vi "HttpGet.vi"() -> ()   [LabVIEW 2016, in "wxpusher.lvlib"]
uses:
  wxpusher.lvlib
  <vilib>/httpClient/LabVIEWHTTPClient.lvlib
panel:
  out "body":string caption="体部"
  out "headers":string caption="头部"
  in  "error in":errorcluster caption="错误输入（无错误）"
  in  "指令+参数":string
  out "结果":string
  out "error out":errorcluster caption="错误输出"
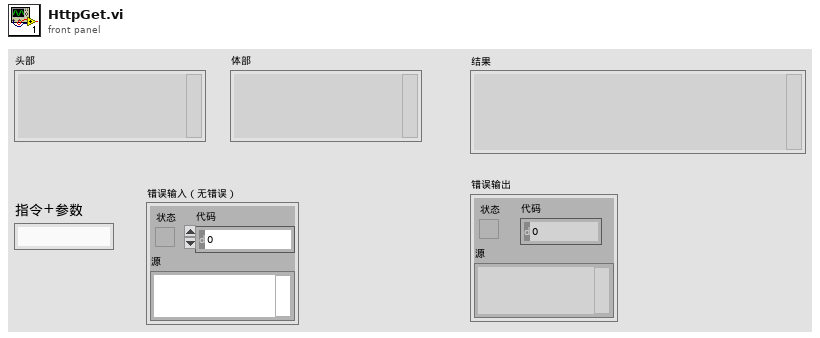
[diagram p1: front panel]
types:
  T1 = typedef "LabVIEWHTTPClient.lvlib/ClientHandle.ctl" = refnum<k1>
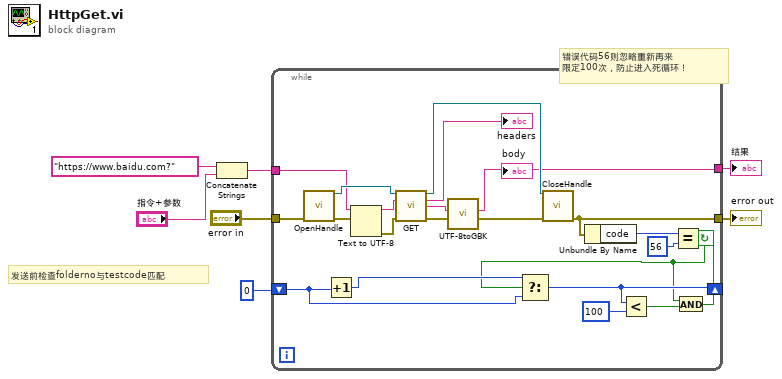
[diagram p0: block diagram]
diagram:
  # "错误代码56则忽略重新再来\n限定100次，防止进入死循环！"
  # "发送前检查folderno与testcode匹配"
  n1 = Concatenate Strings("https://www.baidu.com?" ("url"), "指令+参数") -> (w6:string)
  n2 = while {
    tunnel: w6 -> [w15]
    tunnel: "error in" -> [w26]
    tunnel: [w8] -> w4
    tunnel: [w25] -> w2
    shift-right: [w20] -> _
    shift-left: 0 -> [w21]
    stop <- w16 continue-if-true
    n3 = call <vilib>:"OpenHandle.vi"("error in (no error)"=w26) -> ("client handle out"=w29:T1, "error out"=w14:errorcluster)  [unwired: 13 in]
    n4 = Increment(x=w21) -> (x+1=w22:i32)
    n5 = Text to UTF-8(8:w14, 11:w15) -> (0:w12:errorcluster, 3:w13:string)  [unwired: 1 in]
    n6 = call <vilib>:"GET.vi"("client handle"=w29, "url"=w13, "error in (no error)"=w12) -> ("client handle out"=w27:T1, "headers"=→"headers":string, "body"=w9:string, "error out"=w11:errorcluster)  [unwired: 9 in]
    n7 = call "UTF-8toGBK.vi"("error in"=w11, "UTF-8"=w9) -> ("error out"=w10:errorcluster, "GBK"=w8:string)  [unwired: 8 in]
    "body" <- w8
    n8 = call <vilib>:"CloseHandle.vi"("client handle"=w27, "error in (no error)"=w10) -> ("error out"=w25:errorcluster)  [unwired: 13 in]
    n9 = Unbundle By Name(w25) -> ("code"=w24:i32)
    n10 = Equal?(x=w24, y=56) -> (x = y?=w17:bool)
    n11 = Select(t=w22, s=w17, f=w21) -> (s? t:f=w20:i32)
    n12 = Less?(x=w20, y=100) -> (x < y?=w18:bool)
    n13 = And(x=w17, y=w18) -> (x .and. y?=w16:bool)
  }
  "error out" <- w2
  "结果" <- w4
